vi "appendDevices.vi"(8 "error in (no error)":errorcluster, 10 "DeviceArrayToAppend":refnum<class "DeviceArray.lvclass">, 11 "DeviceArray in":refnum<class "DeviceArray.lvclass">) -> (0 "error out":errorcluster, 3 "DeviceArray out":refnum<class "DeviceArray.lvclass">)   [LabVIEW 2009, in "Tools.lvlib" / "DatabaseHelpers.lvlib" / "DeviceArray.lvclass"]
uses:
  DeviceArray.lvclass
  DeviceArray.lvclass/DeviceArray.ctl
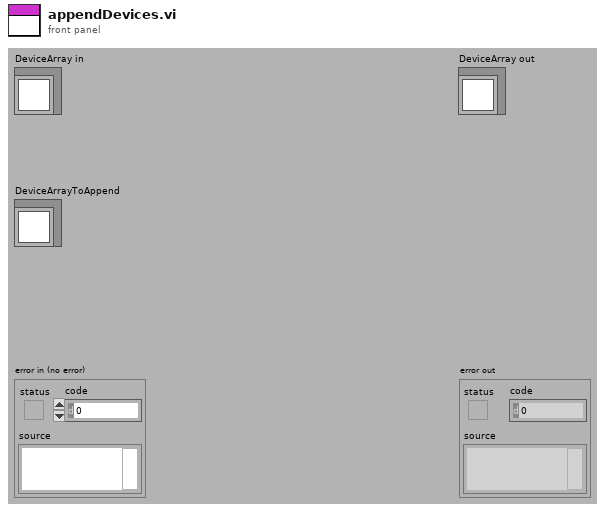
[diagram p1: front panel]
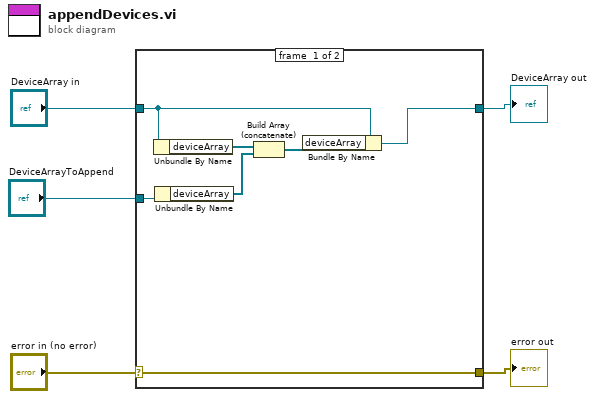
[diagram p0: block diagram]
diagram:
  n1 = case shown="No Error" "error in (no error)" {
    selector: "error in (no error)" -> [w12 w14]
    tunnel: [w12 w14] -> w4
    tunnel: [w6 w13] -> w2
    tunnel: "DeviceArray in" -> [w7 w13]
    tunnel: "DeviceArrayToAppend" -> [w11 _]
    frame #0 {
      n2 = Unbundle By Name(w7) -> ("deviceArray"=w9:refnum<class "device.lvclass">[])
      n3 = Unbundle By Name(w11) -> ("deviceArray"=w10:refnum<class "device.lvclass">[])
      n4 = Build Array (concatenate)(w9, w10) -> (w8:refnum<class "device.lvclass">[])
      n5 = Bundle By Name(cluster=w7, "deviceArray"=w8) -> (w6:refnum<class "DeviceArray.lvclass">)
    }
    frame #1 {
    }
  }
  "error out" <- w4
  "DeviceArray out" <- w2
